vi "weighted average.vi"(3 "weighting":dbl[](array[numeric]), 5 "elements":dbl[](array[numeric])) -> (0 "total weight":dbl, 1 "average":dbl)   [LabVIEW 2009]
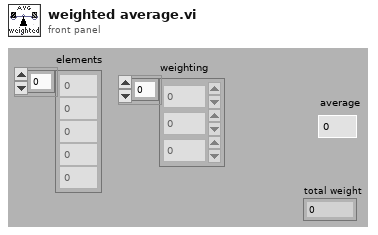
[diagram p1: front panel]
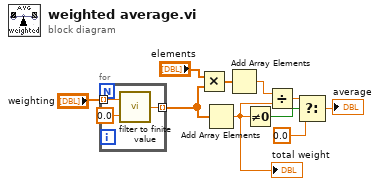
[diagram p0: block diagram]
diagram:
  n1 = for {
    tunnel: [w13] -> w2 mode=indexing
    tunnel: "weighting" -> [w12] mode=indexing
    n2 = call "filter to finite value.vi"("replacement value"=0.0, "value"=w12) -> ("filtered value"=w13:dbl)  [unwired: 1 in]
  }
  n3 = Multiply(x="elements", y=w2) -> (x*y=w9:dbl[])
  n4 = Add Array Elements(numeric array=w2) -> (sum=w7:dbl)
  "total weight" <- w7
  n5 = Add Array Elements(numeric array=w9) -> (sum=w8:dbl)
  n6 = Not Equal To 0?(x=w7) -> (x != 0?=w5:bool)
  n7 = Divide(x=w8, y=w7) -> (x/y=w6:dbl)
  n8 = Select(t=w6, s=w5, f=0.0) -> (s? t:f=→"average":dbl)
